vi "PhaseConversion.vi"(5 "[O_B]":dbl, 7 "Target Lifetime (s)":dbl, 8 "Mod freq (Hz)":dbl, 9 "[V_DC]":dbl, 10 "Mixer Values":dbl[](array[numeric])) -> (0 "V_IF_min":dbl, 1 "V_IF_max":dbl, 2 "M/B":dbl, 3 "Phase Calibration Curve":dbl[](array[numeric]))   [LabVIEW 2018]
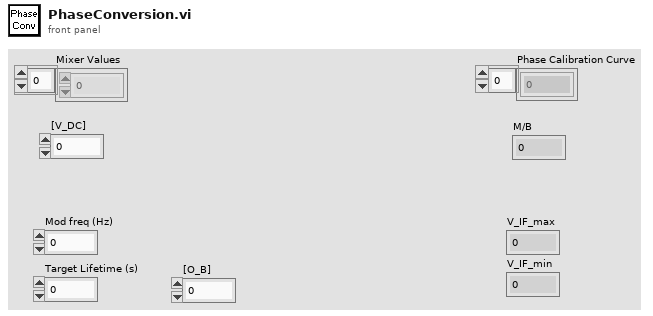
[diagram p1: front panel]
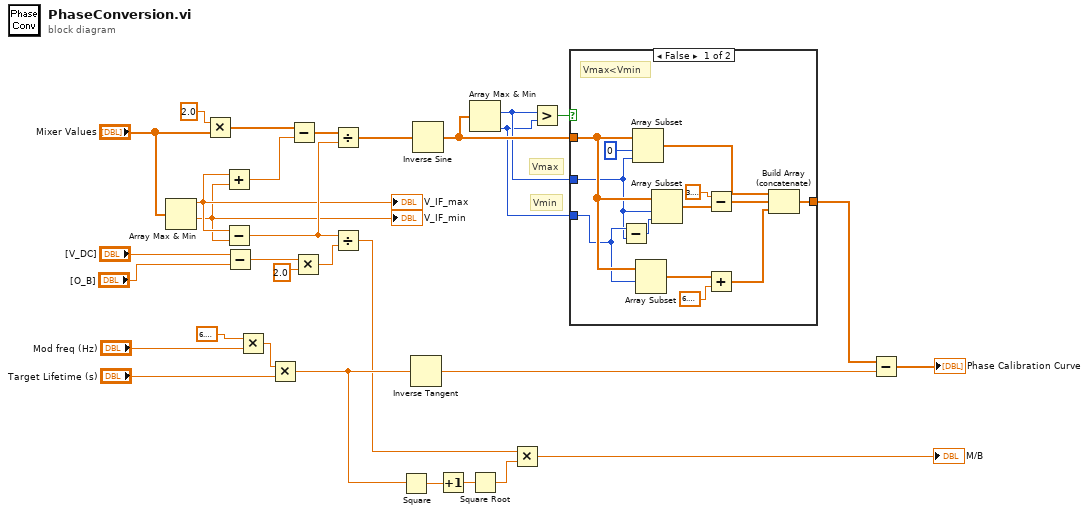
[diagram p0: block diagram]
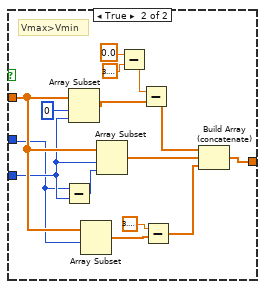
[diagram p2: hidden frame]
diagram:
  # "Vmin"
  # "Vmax"
  n1 = Array Max & Min(array="Mixer Values") -> (max value=w7:dbl, min value=w6:dbl)  [unwired: 2 out]
  "V_IF_max" <- w7
  "V_IF_min" <- w6
  n2 = Multiply(x=2.0 ("y"), y="Mixer Values") -> (x*y=w14:dbl[])
  n3 = Add(x=w7, y=w6) -> (x+y=w11:dbl)
  n4 = Subtract(x=w7, y=w6) -> (x-y=w9:dbl)
  n5 = Subtract(x="[V_DC]", y="[O_B]") -> (x-y=w2:dbl)
  n6 = Multiply(x=6.283185307179586, y="Mod freq (Hz)") -> (x*y=w26:dbl)
  n7 = Multiply(x=w26, y="Target Lifetime (s)") -> (x*y=w20:dbl)
  n8 = Subtract(x=w14, y=w11) -> (x-y=w13:dbl[])
  n9 = Multiply(x=w2, y=2.0) -> (x*y=w1:dbl)
  n10 = Divide(x=w13, y=w9) -> (x/y=w12:dbl[])
  n11 = Divide(x=w9, y=w1) -> (x/y=w8:dbl)
  n12 = Square(x=w20) -> (x^2=w19:dbl)
  n13 = Inverse Tangent(1:w20) -> (0:w22:dbl)
  n14 = Inverse Sine(1:w12) -> (0:w30:dbl[])
  n15 = Increment(x=w19) -> (x+1=w18:dbl)
  n16 = Array Max & Min(array=w30) -> (max index (indices)=w29:i32, min index (indices)=w28:i32)  [unwired: 2 out]
  n17 = Square Root(x=w18) -> (sqrt(x)=w17:dbl)
  n18 = Multiply(x=w8, y=w17) -> (x*y=→"M/B":dbl)
  n19 = Greater?(x=w29, y=w28) -> (0:w31:bool)
  n20 = case shown="False" w31 {
    tunnel: w30 -> [w42 w58]
    tunnel: w28 -> [w34 w47]
    tunnel: w29 -> [w33 w46]
    tunnel: [w35 w48] -> w23
    frame False {
      # "Vmax<Vmin"
      n21 = Subtract(x=w34, y=w33) -> (x-y=w32:i32)
      n22 = Array Subset(array=w42, index=0, length=w33) -> (w41:dbl[])
      n23 = Array Subset(array=w42, index=w34) -> (w38:dbl[])  [unwired: 1 in]
      n24 = Array Subset(array=w42, index=w33, length=w32) -> (w39:dbl[])
      n25 = Subtract(x=3.141592653589793, y=w39) -> (x-y=w40:dbl[])
      n26 = Add(x=w38, y=6.283185307179586) -> (x+y=w36:dbl[])
      n27 = Build Array (concatenate)(w41, w40, w36) -> (w35:dbl[])
    }
    frame True {
      # "Vmax>Vmin"
      n28 = Subtract(x=w46, y=w47) -> (x-y=w45:i32)
      n29 = Array Subset(array=w58, index=0, length=w47) -> (w53:dbl[])
      n30 = Array Subset(array=w58, index=w46) -> (w50:dbl[])  [unwired: 1 in]
      n31 = Array Subset(array=w58, index=w47, length=w45) -> (w57:dbl[])
      n32 = Subtract(x=0.0, y=3.141592653589793) -> (x-y=w54:dbl)
      n33 = Subtract(x=w54, y=w53) -> (x-y=w52:dbl[])
      n34 = Subtract(x=3.141592653589793, y=w50) -> (x-y=w49:dbl[])
      n35 = Build Array (concatenate)(w52, w57, w49) -> (w48:dbl[])
    }
  }
  n36 = Subtract(x=w23, y=w22) -> (x-y=→"Phase Calibration Curve":dbl[])
